vi "Destroy.vi"(8 "error in (no error)":errorcluster, 11 "GenBus_Load_Calculator in":refnum<class "CANBus_Load_Calculator.lvclass">) -> (0 "error out":errorcluster)   [LabVIEW 2018, in "NI-XNET Monitor Engine.lvlib" / "XNET-Bus-Load-Calculator.lvlib" / "CANBus_Load_Calculator.lvclass"]
uses:
  CANBus_Load_Calculator.lvclass
  typedefs/ToCalculator_Data.ctl
  CANBus_Load_Calculator.lvclass/CANBus_Load_Calculator.ctl
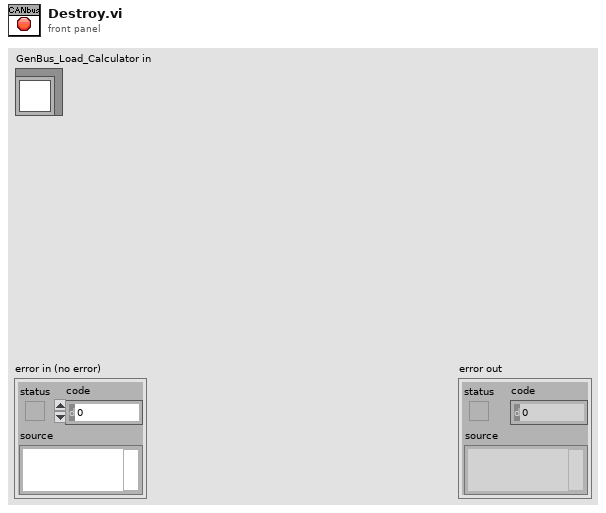
[diagram p1: front panel]
types:
  T1 = typedef "NI-XNET Monitor Engine.lvlib/XNET-Bus-Load-Calculator.lvlib/CANBus_Load_Calculator.lvclass/ToCalculator_Data.ctl" = cluster{"Stop":bool, "Bus Busy Time (us)":u64}
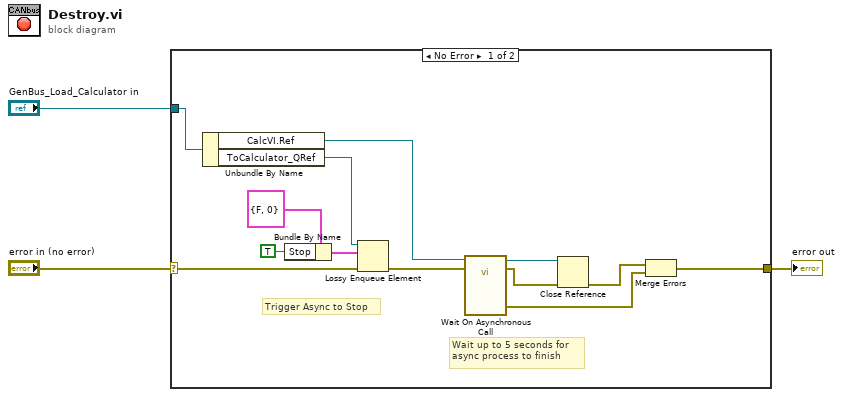
[diagram p0: block diagram]
diagram:
  n1 = case shown="No Error" "error in (no error)" {
    selector: "error in (no error)" -> [w15 w17]
    tunnel: [w4 w17] -> w2
    tunnel: "GenBus_Load_Calculator in" -> [w16 _]
    frame No Error {
      # "Wait up to 5 seconds for \nasync process to finish"
      # "Trigger Async to Stop"
      n2 = Unbundle By Name(w16) -> ("CalcVI.Ref"=w10:refnum<vi>, "ToCalculator_QRef"=w14:refnum<queue>)
      n3 = Bundle By Name(cluster=T1 {"Stop"=FALSE, "Bus Busy Time (us)"=0} ("element"), "Stop"=TRUE) -> (w12:T1)
      n4 = Lossy Enqueue Element(queue=w14, element=w12, error in (no error)=w15) -> (error out=w9:errorcluster)  [unwired: 3 out]
      n5 = call-by-ref "Wait On Asynchronous Call"(reference=w10, error in=w9) -> (reference out=w8:refnum<vi>, error out=w7:errorcluster, 0:"error out"=w5:errorcluster)  [unwired: 11 in]
      n6 = Close Reference(reference=w8, error in (no error)=w7) -> (error out=w6:errorcluster)
      n7 = Merge Errors(w6, w5) -> (w4:errorcluster)
    }
    frame Error {
    }
  }
  "error out" <- w2
